vi "lane_point.vi"(11 "sensor_log_body":dbl[][](array[numeric])) -> ()   [LabVIEW 2012]
uses:
  G_SEN.vi
panel:
  out "appended array":dbl[][](array[numeric])
  out "sensor_log_body 2":dbl[][](array[numeric])
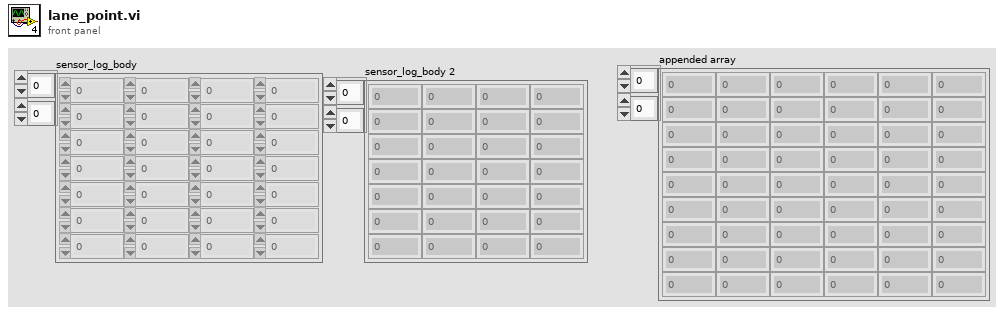
[diagram p1: front panel]
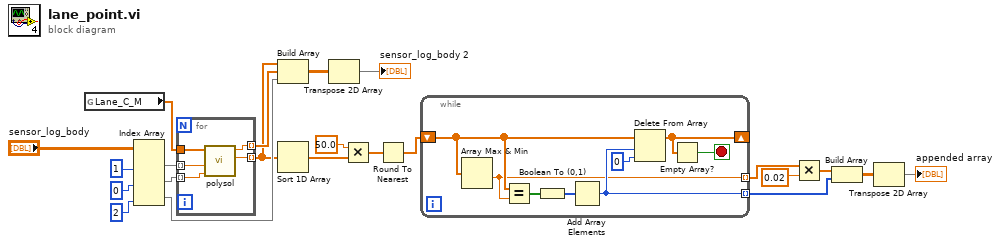
[diagram p0: block diagram]
diagram:
  n1 = global read "G_SEN.vi" "Lane_C_M"() -> (w19:dbl[])
  n2 = Index Array(array="sensor_log_body", index (col) #1=1 ("disabled index (col)"), index (col) #2=0 ("index (col)"), index (col) #3=2 ("index (col)")) -> (element #1=w20:dbl[], element #2=w12:dbl[], element #3=w18:dbl[])  [unwired: 3 in]
  n3 = for {
    tunnel: w20 -> [w27] mode=indexing
    tunnel: w12 -> [w26] mode=indexing
    tunnel: w19 -> [w25]
    tunnel: [w24] -> w15 mode=indexing
    tunnel: [w23] -> w11 mode=indexing
    n4 = call "polysol.vi"("y0"=w26, "x0"=w27, "Lane_C_M"=w25) -> ("Y"=w23:dbl, "X"=w24:dbl)  [unwired: 5 in, 2 out]
  }
  n5 = Build Array(w11, w15, w18) -> (w14:dbl[][])
  n6 = Sort 1D Array(array=w11) -> (sorted array=w10:dbl[])
  n7 = Transpose 2D Array(2D array=w14) -> (transposed array=→"sensor_log_body 2":dbl[][])
  n8 = Multiply(x=50.0, y=w10) -> (x*y=w8:dbl[])
  n9 = Round To Nearest(number=w8) -> (nearest integer value=w7:dbl[])
  n10 = while {
    shift-right: [w29] -> _
    shift-left: w7 -> [w31]
    tunnel: [w32] -> w1 mode=indexing
    tunnel: [w30] -> w6 mode=indexing
    stop <- w28 stop-if-true
    n11 = Array Max & Min(array=w31) -> (min value=w30:dbl)  [unwired: 3 out]
    n12 = Equal?(x=w31, y=w30) -> (x = y?=w35:bool[])
    n13 = Boolean To (0,1)(Boolean=w35) -> (0, 1=w34:i16[])
    n14 = Add Array Elements(numeric array=w34) -> (sum=w32:i16)
    n15 = Delete From Array(array=w31, length=w32, index=0) -> (array with subset deleted=w29:dbl[])  [unwired: 1 out]
    n16 = Empty Array?(array=w29) -> (empty?=w28:bool)
  }
  n17 = Multiply(x=w6, y=0.02) -> (x*y=w2:dbl[])
  n18 = Build Array(w2, w1) -> (w4:dbl[][])
  n19 = Transpose 2D Array(2D array=w4) -> (transposed array=→"appended array":dbl[][])
